vi "Задание_АБ_113.vi"() -> ()   [LabVIEW 2017]
uses:
  <vilib>/Analysis/NI_AALBase.lvlib
  <vilib>/Analysis/1siggen.llb/Ramp Pattern by Samples.vi
panel:
  in  "Циклов в секунду (Модуляция)":i32(slide) scale=0.0..10.0
  out "Цифровой сигнал с паузами 2":dbl[](graph)
  in  "Количесво выборок (сэмплов) в сигнале":i32=1024
  in  "Сколько битов брать":i32=32
  out "Цифровой сигнал с паузами":dbl[](graph)
  out "Массив с паузами":dbl[](array[numeric])
  in  "Количество \nгенерируемых бит":i32=8
  out "Вырезка из массива":dbl[](array[numeric])
  out "Биты на выходе 1":dbl[](array[numeric])
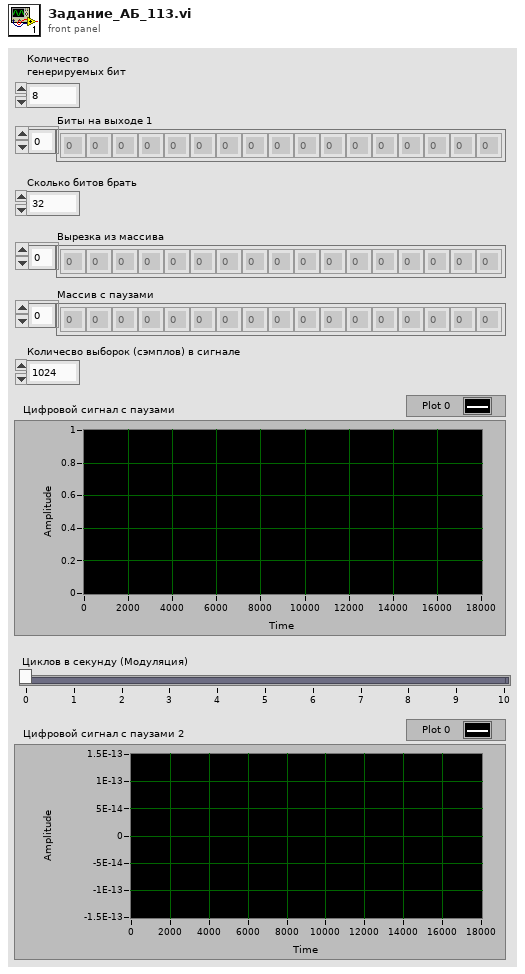
[diagram p1: front panel]
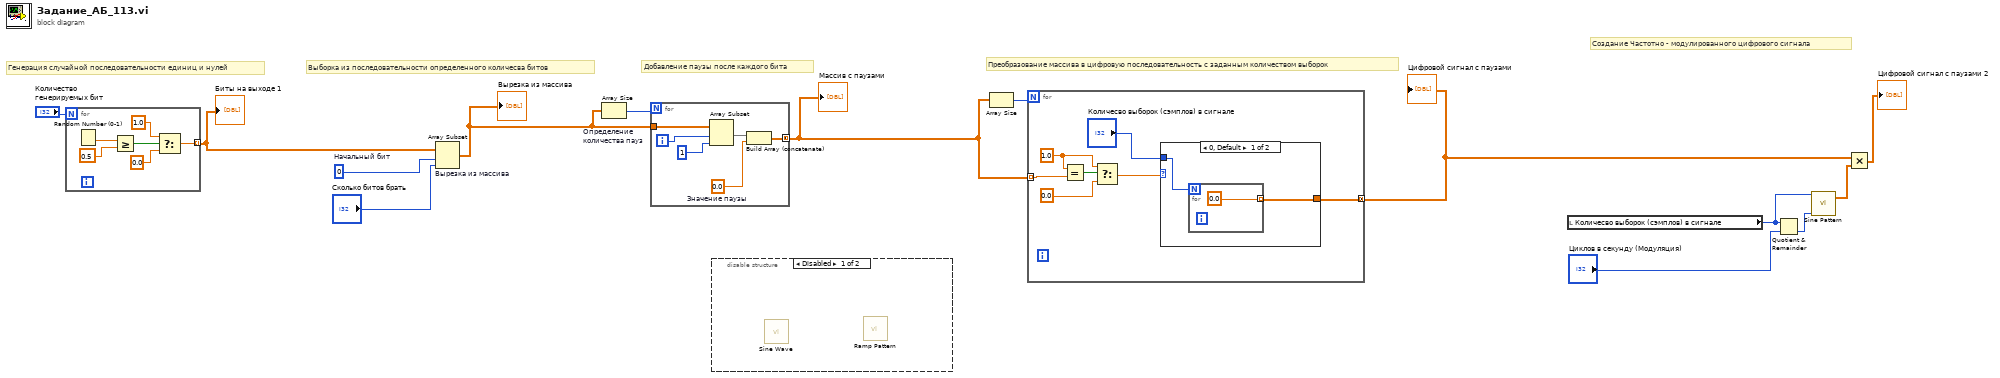
[diagram p0: block diagram]
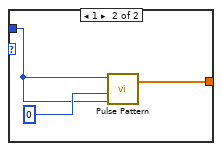
[diagram p2: hidden frame]
diagram:
  w13 = 0  # Начальный бит
  # "Преобразование массива в цифровую последовательность с заданным количеством выборок"
  # "Создание Частотно - модулированного цифрового сигнала"
  # "Добавление паузы после каждого бита"
  # "Выборка из последовательности определенного количесва битов"
  # "Генерация случайной последовательности единиц и нулей"
  n1 = for {
    N: "Количество \nгенерируемых бит" -> [_]
    tunnel: [w15] -> w11 mode=indexing
    n2 = Random Number (0-1)() -> (number: 0 to 1=w20:dbl)
    n3 = Greater Or Equal?(x=w20, y=0.5) -> (x >= y?=w18:bool)
    n4 = Select(t=1.0, s=w18, f=0.0) -> (s? t:f=w15:dbl)
  }
  "Биты на выходе 1" <- w11
  n5 = Array Subset "Вырезка из массива"(array=w11, index=w13, length="Сколько битов брать") -> (w9:dbl[])
  "Вырезка из массива" <- w9
  n6 = Array Size "Определение количества пауз"(array=w9) -> (size(s)=w10:i32)
  n7 = for {
    N: w10 -> [_]
    tunnel: w9 -> [w23]
    tunnel: [w22] -> w8 mode=concatenating
    i -> [w21]
    w24 = 0.0  # Значение паузы
    n8 = Array Subset(array=w23, index=w21, length=1) -> (w25:dbl[])
    n9 = Build Array (concatenate)(w25, w24) -> (w22:dbl[])
  }
  "Массив с паузами" <- w8
  n10 = disable-structure shown="Disabled" {
    frame Disabled {
      n11 = call <vilib>:"Sine Wave.vi"() -> ()  [unwired: 5 in, 3 out]
      n12 = call-poly <vilib>:"Ramp Pattern.vi"() -> ()  [unwired: 10 in, 2 out]
    }
    frame Enabled {
    }
  }
  n13 = Array Size(array=w8) -> (size(s)=w7:i32)
  n14 = for {
    N: w7 -> [_]
    tunnel: w8 -> [w30] mode=indexing
    tunnel: [w28] -> w4 mode=concatenating
    w32 = 1.0
    n15 = Equal?(x=w32, y=w30) -> (x = y?=w33:bool)
    n16 = Select(t=w32, s=w33, f=0.0) -> (s? t:f=w29:dbl)
    n17 = case shown="0, Default" w29 {
      tunnel: [w34 w38] -> w28
      tunnel: "Количесво выборок (сэмплов) в сигнале" -> [w35 w37]
      frame 0, Default {
        n18 = for {
          N: w35 -> [_]
          tunnel: [0.0] -> w34 mode=indexing
        }
      }
      frame 1 {
        n19 = call <vilib>:"Pulse Pattern.vi"("width"=w37, "delay"=0, "samples"=w37) -> ("Pulse Pattern"=w38:dbl[])  [unwired: 1 in, 1 out]
      }
    }
  }
  "Цифровой сигнал с паузами" <- w4
  n20 = local read "Количесво выборок (сэмплов) в сигнале"() -> (w3:i32)
  n21 = Quotient & Remainder(x=w3, y="Циклов в секунду (Модуляция)") -> (floor(x/y)=w5:i32)  [unwired: 1 out]
  n22 = call <vilib>:"Sine Pattern.vi"("cycles"=w5, "samples"=w3) -> ("Sinusoidal Pattern"=w6:dbl[])  [unwired: 2 in, 1 out]
  n23 = Multiply(x=w4, y=w6) -> (x*y=→"Цифровой сигнал с паузами 2":dbl[])
